vi "testConfigServer.vi"(8 "error in (no error)":errorcluster) -> (0 "error out":errorcluster)   [LabVIEW 2018]
doc: "Test the configServer.vi."
uses:
  src/TcpServer/TcpServer.lvclass
  src/TcpServerTel/typedef/enqueueOptionsTypeDef.ctl
  src/TcpServer/TcpServer.lvclass/TcpServer.ctl
  src/TcpServerBase/TcpServerBase.lvclass/TcpServerBase.ctl
  src/TcpServerTel/TcpServerTel.lvclass/TcpServerTel.ctl
  src/TcpServerCmd/TcpServerCmd.lvclass
  home/pcortes/github/ts_labview_tcp_json/src/TcpServerBase/TcpServerBase.lvclass
  src/TcpServerTel/TcpServerTel.lvclass
  <vilib>/addons/_JKI Toolkits/Caraya/classes/Assert/Assert Not Equal Value_Variant.vi
  <vilib>/addons/_JKI Toolkits/Caraya/classes/Assert/Assert Equal Value_Variant.vi
  <vilib>/addons/_JKI Toolkits/Caraya/classes/Test/Test.lvclass
  <vilib>/addons/_JKI Toolkits/Caraya/classes/Assert/Assert.lvclass
  src/TcpServerBase/TcpServerBase.lvclass
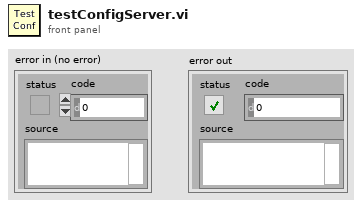
[diagram p1: front panel]
types:
  T1 = typedef "TcpServerTel.lvclass/enqueueOptionsTypeDef.ctl" = enum16{"lossy enqueue", "normal enqueue"}
  T2 = cluster{"cmdServerPort":u16, "telServerPort":u16, "serverTimeout (ms)":i32, "serverBytesToRead":i32, "queueTcpClientFromDdsMaxSize":i32, "EnqueueOptions":T1, "timeoutQueueTel (ms)":i32, "queueTcpClientMaxSize":i32, "timeoutInMs":i32}
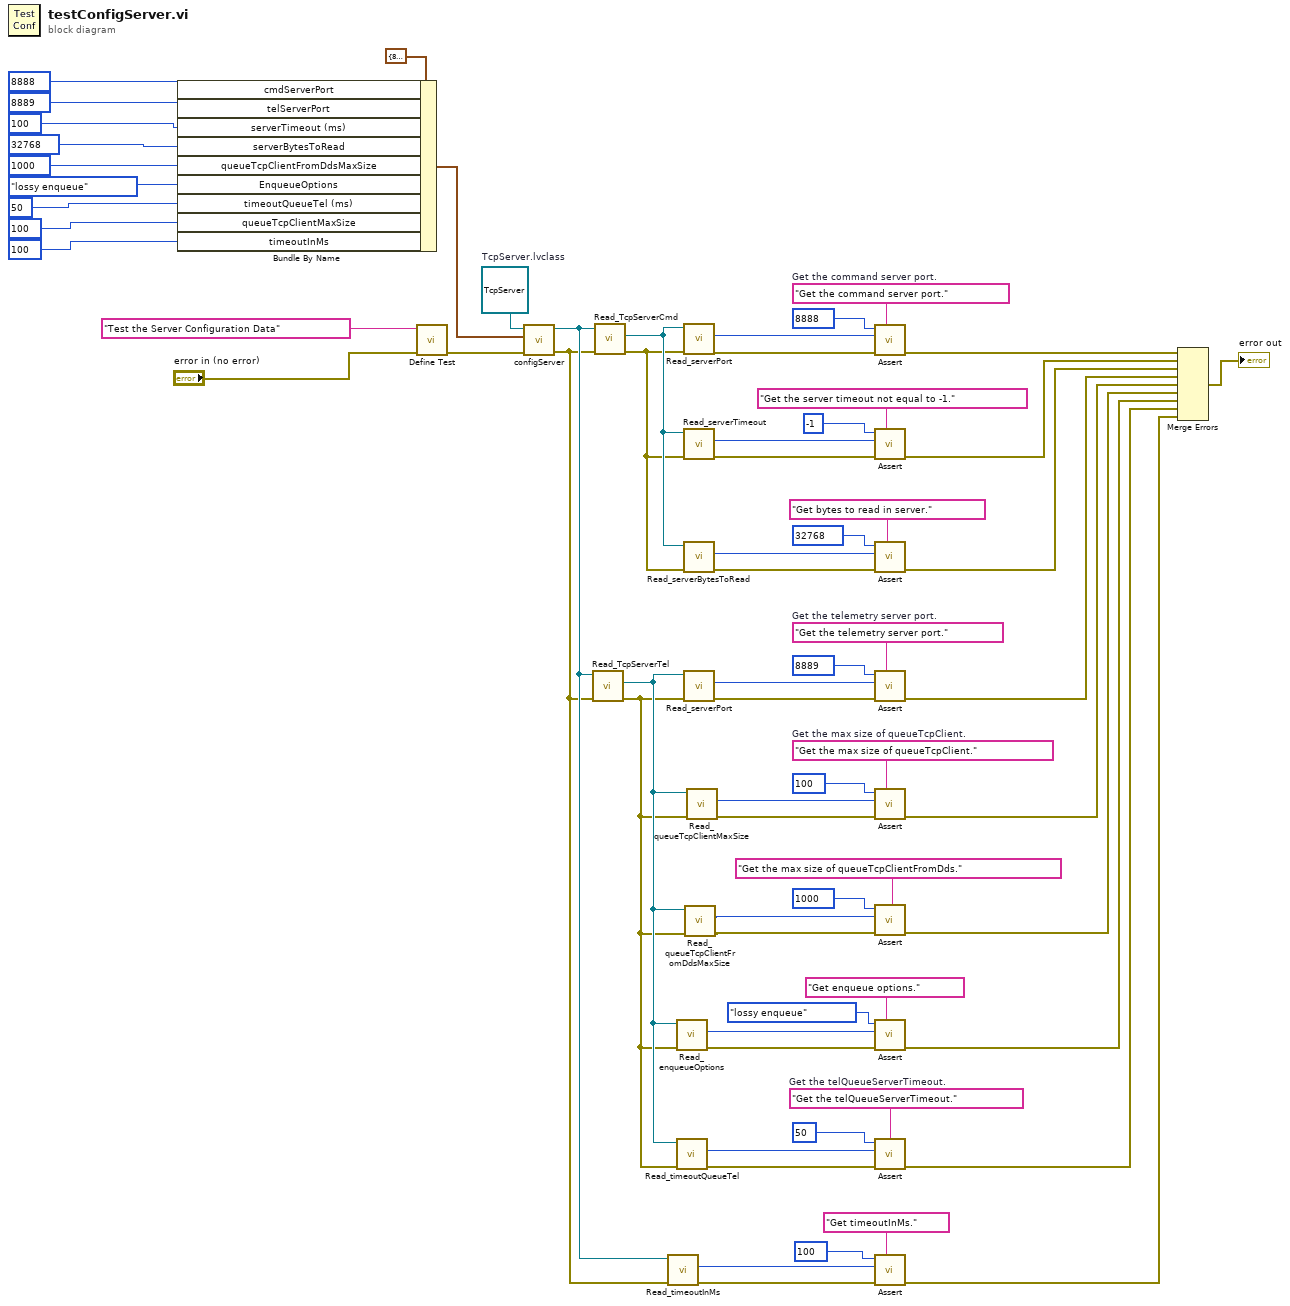
[diagram p0: block diagram]
diagram:
  w37 = "Get the max size of queueTcpClient."  # Get the max size of queueTcpClient.
  w40 = "Get the telQueueServerTimeout."  # Get the telQueueServerTimeout.
  w47 = "Get the telemetry server port."  # Get the telemetry server port.
  w53 = refnum<class "TcpServer.lvclass"> refnum  # TcpServer.lvclass
  w63 = "Get the command server port."  # Get the command server port.
  n1 = Bundle By Name(cluster=T2 {"cmdServerPort"=8888, "telServerPort"=8889, "serverTimeout (ms)"=100, "serverBytesToRead"=32768, "queueTcpClientFromDdsMaxSize"=5, "EnqueueOptions"=enum."lossy enqueue", "timeoutQueueTel (ms)"=50, "queueTcpClientMaxSize"=1000, "timeoutInMs"=100} ("ServerConfiguration"), "cmdServerPort"=u16 8888, "telServerPort"=u16 8889, "serverTimeout (ms)"=100, "serverBytesToRead"=32768, "queueTcpClientFromDdsMaxSize"=1000 ("telQueueServerMaxSize"), "EnqueueOptions"=enqueueOptionsTypeDef."lossy enqueue", "timeoutQueueTel (ms)"=50 ("telQueueServerTimeout"), "queueTcpClientMaxSize"=100 ("tcpClientQueueMaxSize"), "timeoutInMs"=100 ("timeoutStatusNotifier")) -> (w2:T2)
  n2 = call <vilib>:"Define Test.vi"("error in (no error)"="error in (no error)", "Label (VI Title)"="Test the Server Configuration Data") -> ("error out"=w65:errorcluster)  [unwired: 9 in]
  n3 = call "configServer.vi"("error in (no error)"=w65, "ServerConfiguration"=w2, "tcpServer in"=w53) -> ("error out"=w12:errorcluster, "tcpServer out"=w13:refnum<class "TcpServer.lvclass">)  [unwired: 7 in]
  n4 = call "Read_TcpServerTel.vi"("error in (no error)"=w12, "TcpServer in"=w13) -> ("error out"=w4:errorcluster, "TcpServerTel.lvclass"=w5:refnum<class "TcpServerTel.lvclass">)  [unwired: 7 in, 1 out]
  n5 = call "Read_TcpServerCmd.vi"("error in (no error)"=w12, "TcpServer in"=w13) -> ("error out"=w7:errorcluster, "TcpServerCmd.lvclass"=w8:refnum<class "TcpServerCmd.lvclass">)  [unwired: 7 in, 1 out]
  n6 = call "Read_timeoutInMs.vi"("error in (no error)"=w12, "TcpServer in"=w13) -> ("error out"=w11:errorcluster, "timeoutInMs"=w10:i32)  [unwired: 7 in, 1 out]
  n7 = call "Read_enqueueOptions.vi"("error in (no error)"=w4, "TcpServerTel in"=w5) -> ("error out"=w32:errorcluster, "EnqueueOptions"=w31:T1)  [unwired: 7 in, 1 out]
  n8 = call "Read_timeoutQueueTel.vi"("error in (no error)"=w4, "TcpServerTel in"=w5) -> ("error out"=w30:errorcluster, "timeoutQueueTel"=w29:i32)  [unwired: 7 in, 1 out]
  n9 = call "Read_serverPort.vi"("error in (no error)"=w7, "TcpServerBase in"=w8) -> ("error out"=w62:errorcluster, "serverPort"=w61:u16)  [unwired: 7 in, 1 out]
  n10 = call "Read_serverTimeout.vi"("error in (no error)"=w7, "TcpServerBase in"=w8) -> ("error out"=w57:errorcluster, "serverTimeout"=w58:i32)  [unwired: 7 in, 1 out]
  n11 = call "Read_serverBytesToRead.vi"("error in (no error)"=w7, "TcpServerBase in"=w8) -> ("error out"=w50:errorcluster, "serverBytesToRead"=w49:i32)  [unwired: 7 in, 1 out]
  n12 = call "Read_serverPort.vi"("error in (no error)"=w4, "TcpServerBase in"=w5) -> ("error out"=w45:errorcluster, "serverPort"=w44:u16)  [unwired: 7 in, 1 out]
  n13 = call "Read_queueTcpClientFromDdsMaxSize.vi"("error in (no error)"=w4, "TcpServerTel in"=w5) -> ("error out"=w34:errorcluster, "queueTcpClientFromDdsMaxSize"=w33:i32)  [unwired: 7 in, 1 out]
  n14 = call "Read_queueTcpClientMaxSize.vi"("error in (no error)"=w4, "TcpServerBase in"=w5) -> ("error out"=w36:errorcluster, "queueTcpClientMaxSize"=w35:i32)  [unwired: 7 in, 1 out]
  n15 = call-poly <vilib>:"Assert.vi"("Label"=w63, "error in (no error)"=w62, "Y"=w61, "X"=8888) -> ("error out"=w56:errorcluster)  [unwired: 7 in]
  n16 = call-poly <vilib>:"Assert.vi"("Label"="Get the server timeout not equal to -1.", "error in (no error)"=w57, "Y"=w58, "X"=-1) -> ("error out"=w55:errorcluster)  [unwired: 7 in]
  n17 = call-poly <vilib>:"Assert.vi"("Label"="Get bytes to read in server.", "error in (no error)"=w50, "Y"=w49, "X"=32768) -> ("error out"=w48:errorcluster)  [unwired: 7 in]
  n18 = call-poly <vilib>:"Assert.vi"("Label"=w47, "error in (no error)"=w45, "Y"=w44, "X"=8889) -> ("error out"=w6:errorcluster)  [unwired: 7 in]
  n19 = call-poly <vilib>:"Assert.vi"("Label"=w37, "error in (no error)"=w36, "Y"=w35, "X"=100) -> ("error out"=w28:errorcluster)  [unwired: 7 in]
  n20 = call-poly <vilib>:"Assert.vi"("Label"="Get the max size of queueTcpClientFromDds.", "error in (no error)"=w34, "Y"=w33, "X"=1000) -> ("error out"=w27:errorcluster)  [unwired: 7 in]
  n21 = call-poly <vilib>:"Assert.vi"("Label"="Get enqueue options.", "error in (no error)"=w32, "Y"=w31, "X"=enqueueOptionsTypeDef."lossy enqueue" ("EnqueueOptions")) -> ("error out"=w26:errorcluster)  [unwired: 7 in]
  n22 = call-poly <vilib>:"Assert.vi"("Label"=w40, "error in (no error)"=w30, "Y"=w29, "X"=50) -> ("error out"=w25:errorcluster)  [unwired: 7 in]
  n23 = call-poly <vilib>:"Assert.vi"("Label"="Get timeoutInMs.", "error in (no error)"=w11, "Y"=w10, "X"=100) -> ("error out"=w3:errorcluster)  [unwired: 7 in]
  n24 = Merge Errors(w56, w55, w48, w6, w28, w27, w26, w25, w3) -> (→"error out":errorcluster)
